vi "KillThreads.vi"(8 "error in (no error)":errorcluster, 11 "Member_Actor in":refnum<class "Member_Actor.lvclass">) -> (0 "error out":errorcluster, 3 "Member_Actor out":refnum<class "Member_Actor.lvclass">)   [LabVIEW 2015, in "Member_Actor.lvlib" / "Member_Actor.lvclass"]
uses:
  Member_Actor.lvclass
  Member_Actor.lvclass/Member_Actor.ctl
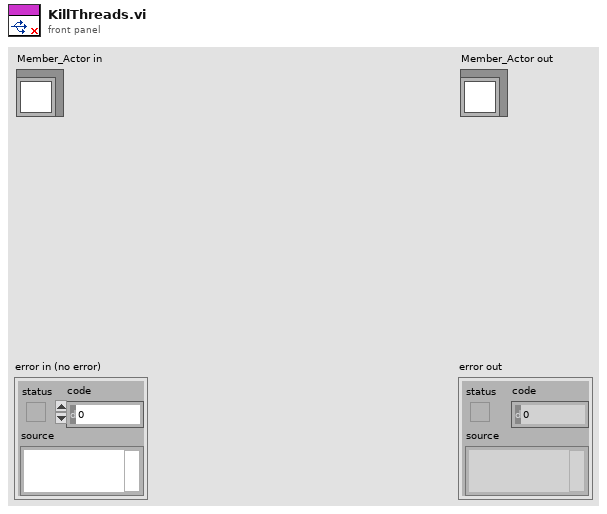
[diagram p1: front panel]
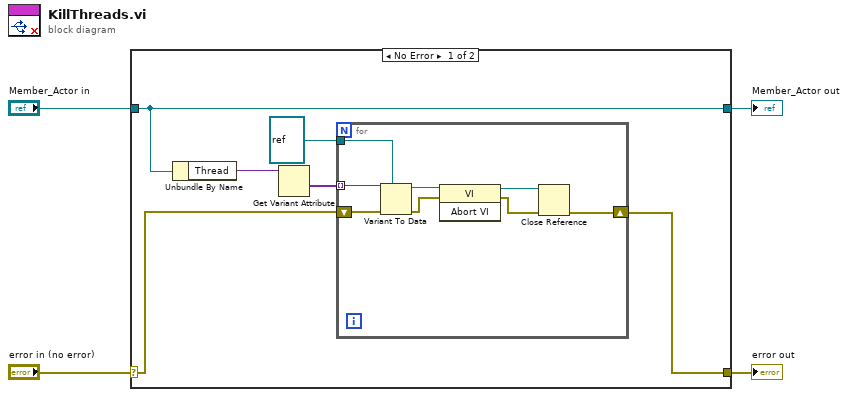
[diagram p0: block diagram]
diagram:
  n1 = case shown="No Error" "error in (no error)" {
    selector: "error in (no error)" -> [w6 w20]
    tunnel: [w5 w20] -> w3
    tunnel: [w10 w19] -> w1
    tunnel: "Member_Actor in" -> [w10 w19]
    frame No Error {
      n2 = Unbundle By Name(w10) -> ("Thread"=w9:variant)
      n3 = Get Variant Attribute(Variant=w9) -> (values=w8:variant[])  [unwired: 3 in, 3 out]
      n4 = for {
        tunnel: w8 -> [w18] mode=indexing
        tunnel: refnum<vi> refnum ("VI Ref") -> [w17]
        shift-right: [w11] -> w5
        shift-left: w6 -> [w16]
        n5 = Variant To Data(error in=w16, type=w17, Variant=w18) -> (data=w15:refnum<vi>, error out=w14:errorcluster)
        n6 = invoke class="VI" method="Abort VI"(reference=w15, error in=w14) -> (reference out=w12:refnum<vi>, error out=w13:errorcluster)  [unwired: 1 in, 1 out]
        n7 = Close Reference(reference=w12, error in (no error)=w13) -> (error out=w11:errorcluster)
      }
    }
    frame Error {
    }
  }
  "error out" <- w3
  "Member_Actor out" <- w1
